vi "GTH.ADC.vi"(4 "Signal Filter":T1, 5 "Error":dbl, 6 "SampleRate":u32=250000 min=1000 max=250000 step=1000, 7 "Rate":dbl=1.0, 8 "Error In":errorcluster caption="错误输入", 9 "Points(X*5k)":u8=1 min=1 max=100, 10 "Channel":enum16{"Channel A", "Channel B"}(ring), 11 "VISA资源输入":refnum<visa-resource-name>) -> (0 "Error Out":errorcluster caption="错误输出", 1 "波形图":waveform(dbl)(graph), 2 "DataOut":T2, 3 "OK?":bool)   [LabVIEW 2012, in "Lib_UEL.ATE.lvlib" / "STM32-CoreBD.lvlib"]
uses:
  STM32-CoreBD.lvlib
  <vilib>/measure/madcrms.llb/Basic Averaged DC-RMS for 1 Chan.vi
  <vilib>/measure/NI_MAPro.lvlib
panel:
  # "Version History\nV01,2015-2-10, 初始版本.\nV02 - 2015-5-25, LIGUANG, 增加滤波选项输出。滤波只针对AC波形及AC有效值。"
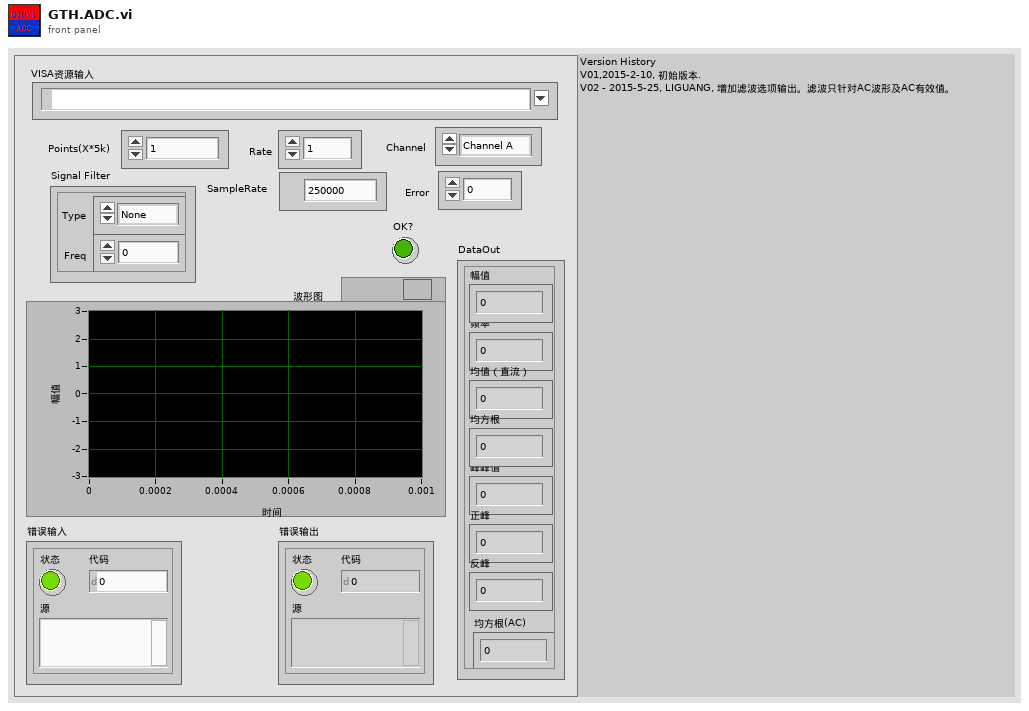
[diagram p1: front panel]
types:
  T1 = cluster{"Type":enum16{"None", "Low Pass", "High Pass"}, "Freq":dbl}
  T2 = cluster{"频率":dbl, "峰峰值":dbl, "均值（直流）":dbl, "均方根":dbl, "正峰":dbl, "反峰":dbl, "幅值":dbl, "均方根(AC)":dbl}
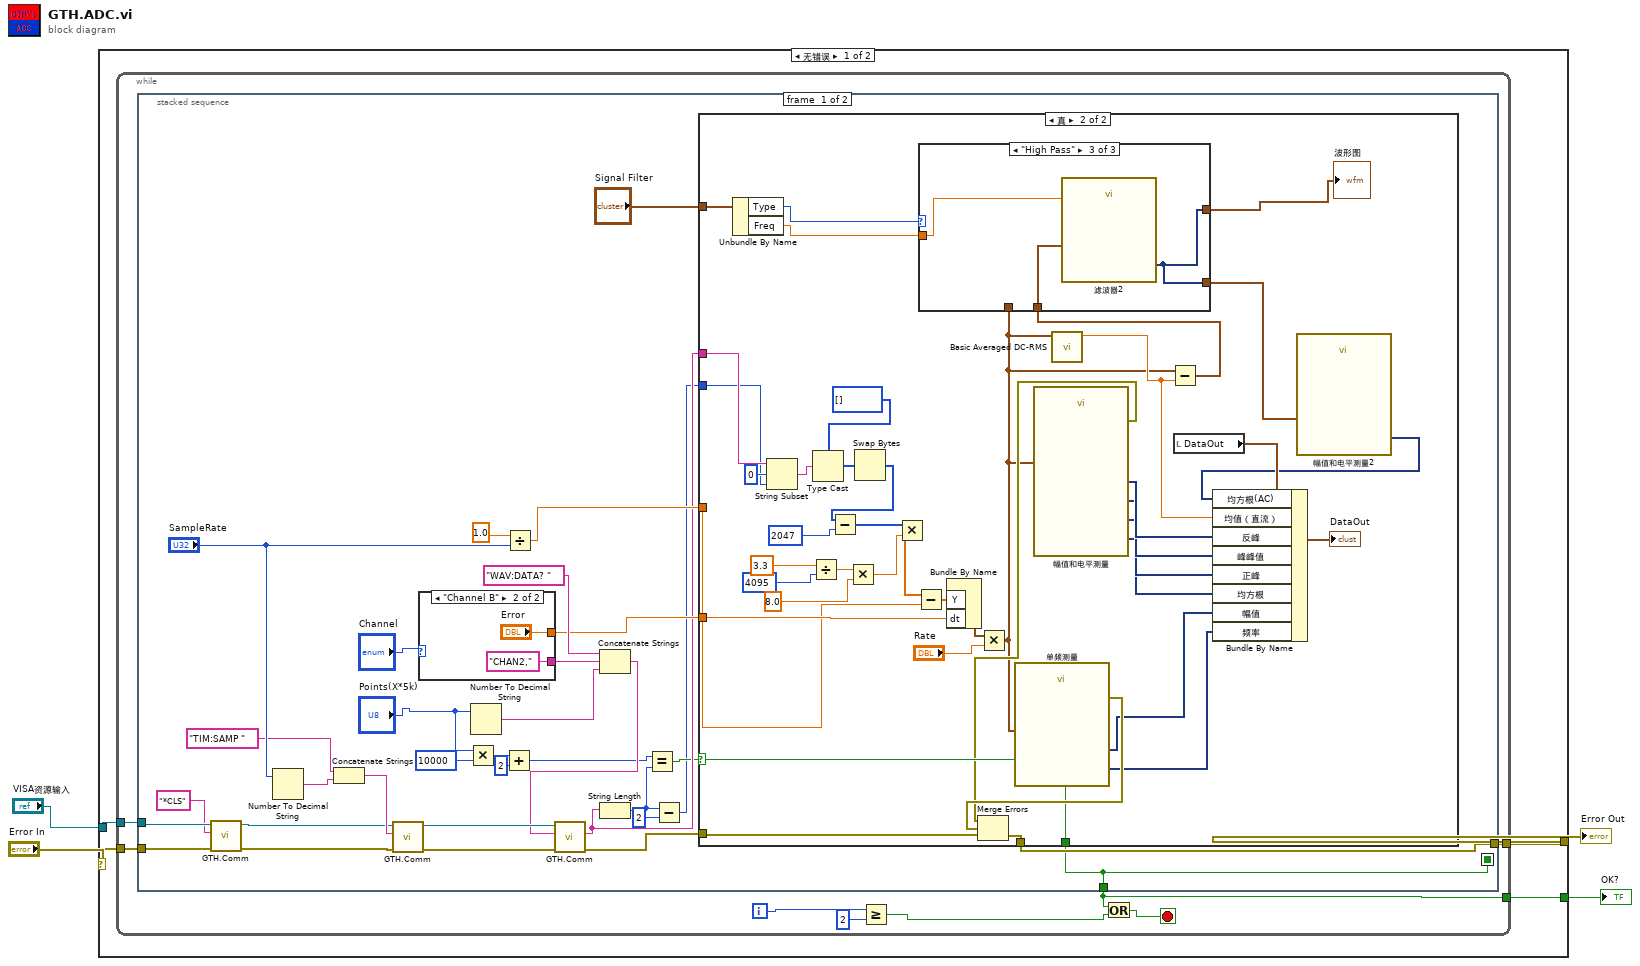
[diagram p0: block diagram]
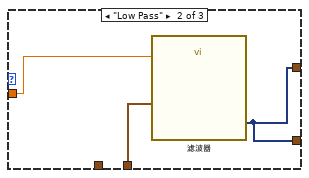
[diagram p4: hidden frame]
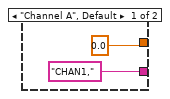
[diagram p5: hidden frame]
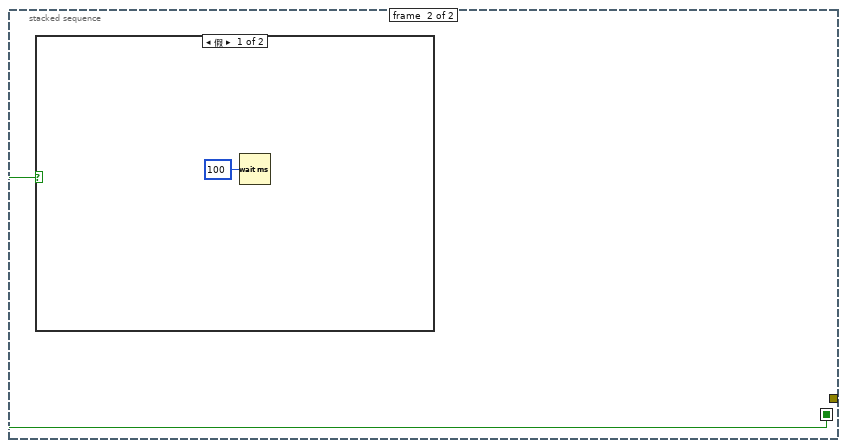
[diagram p6: hidden frame]
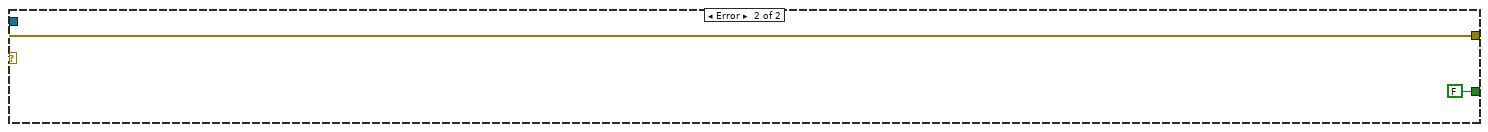
[diagram p8: hidden frame]
diagram:
  n1 = case shown="无错误" "Error In" {
    selector: "Error In" -> [w6 w109]
    tunnel: [w8 w109] -> w2
    tunnel: "VISA资源输入" -> [w7 _]
    tunnel: [w5 FALSE] -> w1
    frame No Error {
      n2 = while {
        tunnel: [w13] -> w8
        tunnel: w7 -> [w16]
        tunnel: w6 -> [w15]
        tunnel: [w9] -> w5
        i -> [w12]
        stop <- w14 stop-if-true
        n3 = stacked-sequence {
          seq-local: [w18 _] -> [_ w106]
          tunnel: w16 -> [w43 _]
          tunnel: w15 -> [w42 _]
          tunnel: [w19 _] -> w13
          tunnel: [w18 _] -> w9
          frame #0 {
            n4 = call "GTH.Comm.vi"("Error In"=w42, "SCPI CMD"="*CLS" ("字符串"), "USB Port In"=w43) -> ("Error Out"=w35:errorcluster, "USB Port Out"=w36:refnum<visa-resource-name>)  [unwired: 3 in, 4 out]
            n5 = Number To Decimal String(number="SampleRate") -> (decimal integer string=w38:string)  [unwired: 1 in]
            n6 = Concatenate Strings("TIM:SAMP " ("字符串"), w38) -> (w37:string)
            n7 = call "GTH.Comm.vi"("Error In"=w35, "SCPI CMD"=w37, "USB Port In"=w36) -> ("Error Out"=w32:errorcluster, "USB Port Out"=w33:refnum<visa-resource-name>)  [unwired: 3 in, 4 out]
            n8 = case shown="\"Channel B\"" "Channel" {
              tunnel: ["CHAN1," ("字符串") "CHAN2," ("字符串")] -> w47
              tunnel: [0.0 "Error"] -> w44
              frame "Channel A", Default {
              }
              frame "Channel B" {
              }
            }
            n9 = Multiply(x="Points(X*5k)", y=u32 10000) -> (x*y=w27:u32)
            n10 = Number To Decimal String(number="Points(X*5k)") -> (decimal integer string=w34:string)  [unwired: 1 in]
            n11 = Add(x=w27, y=u32 2) -> (x+y=w24:u32)
            n12 = Divide(x=1.0 ("y"), y="SampleRate") -> (x/y=w45:dbl)
            n13 = Concatenate Strings("WAV:DATA? " ("字符串"), w47, w34) -> (w31:string)
            n14 = call "GTH.Comm.vi"("Error In"=w32, "SCPI CMD"=w31, "USB Port In"=w33) -> ("Error Out"=w30:errorcluster, "Return"=w25:string)  [unwired: 3 in, 4 out]
            n15 = String Length(string=w25) -> (length=w22:i32)
            n16 = Equal?(x=w24, y=w22) -> (x = y?=w23:bool)
            n17 = Subtract(x=w22, y=2) -> (x-y=w20:i32)
            n18 = case shown="真" w23 {
              selector: w23 -> [w50 w65]
              tunnel: w45 -> [_ w85]
              tunnel: [w51 w77] -> w19
              tunnel: w44 -> [_ w71]
              tunnel: w30 -> [w51 w70]
              tunnel: w25 -> [_ w68]
              tunnel: w20 -> [_ w66]
              tunnel: [w50 w65] -> w18
              tunnel: "Signal Filter" -> [_ w58]
              frame False {
              }
              frame True {
                n19 = Unbundle By Name(w58) -> ("Type"=w57:enum16{"None", "Low Pass", "High Pass"}, "Freq"=w52:dbl)
                n20 = String Subset(string=w68, offset (0)=0 ("偏移量(0)"), length (rest)=w66) -> (substring=w69:string)
                n21 = Divide(x=3.3 ("y"), y=4095 ("偏移量(0)")) -> (x/y=w89:dbl)
                n22 = Type Cast(type=u16[] [], x=w69) -> (*(type *) &x=w92:u16[])
                n23 = Multiply(x=w89, y=8.0) -> (x*y=w86:dbl)
                n24 = Swap Bytes(anything=w92) -> (byte swapped=w91:u16[])
                n25 = Subtract(x=w91, y=2047 ("偏移量(0)")) -> (x-y=w87:i32[])
                n26 = Multiply(x=w87, y=w86) -> (x*y=w72:dbl[])
                n27 = Subtract(x=w72, y=w71) -> (x-y=w73:dbl[])
                n28 = Bundle By Name("Y"=w73, "dt"=w85) -> (w76:waveform(dbl))  [unwired: 1 in]
                n29 = Multiply(x=w76, y="Rate") -> (x*y=w55:waveform(dbl))
                n30 = call "单频测量"("Signals"=w55) -> ("error out"=w82:errorcluster, "Frequency"=w78:dynamicdata, "Amplitude"=w79:dynamicdata)  [unwired: 8 in]
                n31 = call "幅值和电平测量"("Signals"=w55) -> ("RMS"=w61:dynamicdata, "Negative Peak"=w64:dynamicdata, "Positive Peak"=w62:dynamicdata, "Peak to Peak"=w63:dynamicdata, "error out"=w59:errorcluster)  [unwired: 10 in]
                n32 = Merge Errors(w59, w82, w70) -> (w77:errorcluster)
                n33 = call-poly <vilib>:"Basic Averaged DC-RMS.vi"("signal in"=w55) -> ("DC value"=w74:dbl)  [unwired: 7 in, 3 out]
                n34 = Subtract(x=w55, y=w74) -> (x-y=w54:waveform(dbl))
                n35 = case shown="\"High Pass\"" w57 {
                  tunnel: [w95 w96 w99] -> w56
                  tunnel: w55 -> [w95 _ _]
                  tunnel: [w94 w96 w99] -> w53
                  tunnel: w54 -> [w94 w98 w101]
                  tunnel: w52 -> [_ w97 w100]
                  frame "None", Default {
                  }
                  frame "Low Pass" {
                    n36 = call "滤波器"("Lower Cut-Off"=w97, "Signal"=w98) -> ("Filtered Signal"=w96:dynamicdata)  [unwired: 8 in, 1 out]
                  }
                  frame "High Pass" {
                    n37 = call "滤波器2"("Lower Cut-Off"=w100, "Signal"=w101) -> ("Filtered Signal"=w99:dynamicdata)  [unwired: 8 in, 1 out]
                  }
                }
                "波形图" <- w56
                n38 = local read "DataOut"() -> (w80:T2)
                n39 = call "幅值和电平测量2"("Signals"=w53) -> ("RMS"=w60:dynamicdata)  [unwired: 13 in, 1 out]
                n40 = Bundle By Name(cluster=w80, "均方根(AC)"=w60, "均值（直流）"=w74, "反峰"=w64, "峰峰值"=w63, "正峰"=w62, "均方根"=w61, "幅值"=w79, "频率"=w78) -> (→"DataOut":T2)
              }
            }
          }
          frame #1 {
            n41 = case shown="假" w106 {
              frame False {
                n42 = Wait (ms)(milliseconds to wait=u32 100 ("等待时间（毫秒）")) -> ()  [unwired: 1 out]
              }
              frame True {
              }
            }
          }
        }
        n43 = Greater Or Equal?(x=w12, y=2) -> (x >= y?=w10:bool)
        n44 = Or(x=w9, y=w10) -> (x .or. y?=w14:bool)
      }
    }
    frame Error {
    }
  }
  "Error Out" <- w2
  "OK?" <- w1
